vi "ESP32 BLE Client.vi"() -> ()   [LabVIEW 2016]
panel:
  in  "Stop":bool
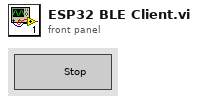
[diagram p1: front panel]
types:
  T1 = cluster{"self":string, "handle":string, "bdaddr":string}[]
  T2 = cluster{"self":string, "handle":string, "bdaddr":string}
  T3 = typedef "BLE reference.ctl" = cluster{"BLE Gateway Base URL":string, "Variant":variant, "Node Address":string}
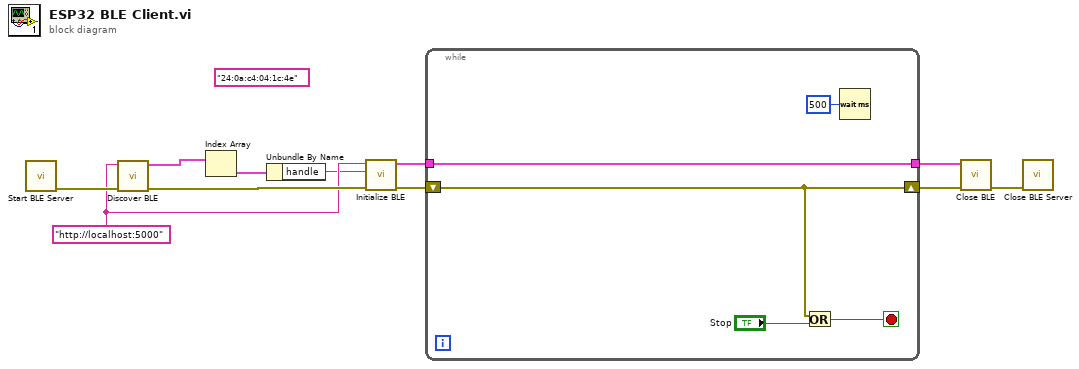
[diagram p0: block diagram]
diagram:
  (unwired) "24:0a:c4:04:1c:4e" ("Node ID")
  w6 = "http://localhost:5000" ("BLE Gateway Base URL")
  n1 = call "Start BLE Server.vi"() -> ("Error Out"=w11:errorcluster)  [unwired: 11 in]
  n2 = call <userlib>:"Discover BLE.vi"("error in (no error)"=w11, "BLE Gateway Base URL"=w6) -> ("error out"=w7:errorcluster, "Nodes"=w10:T1)  [unwired: 8 in]
  n3 = Index Array(array=w10) -> (element=w9:T2)  [unwired: 1 in]
  n4 = Unbundle By Name(w9) -> ("handle"=w1:string)
  n5 = call <userlib>:"Initialize BLE.vi"("error in (no error)"=w7, "Node ID"=w1, "BLE Gateway Base URL"=w6) -> ("error out"=w8:errorcluster, "BLE reference out"=w5:T3)  [unwired: 7 in]
  n6 = while {
    shift-right: [w13] -> w4
    shift-left: w8 -> [w13]
    tunnel: w5 -> [w12]
    tunnel: [w12] -> w3
    stop <- w14 stop-if-true
    n7 = Or(x=w13, y="Stop") -> (x .or. y?=w14:bool)
    n8 = Wait (ms)(milliseconds to wait=u32 500) -> ()  [unwired: 1 out]
  }
  n9 = call <userlib>:"Close BLE.vi"("error in (no error)"=w4, "BLE reference in"=w3) -> ("error out"=w2:errorcluster)  [unwired: 9 in]
  n10 = call "Close BLE Server.vi"("Error In"=w2) -> ()  [unwired: 10 in, 1 out]
